vi "Server Client Loop.vi"(0 "Local Hash":string, 3 "Event Logging":refnum<class "EventLoggingService.lvclass">, 4 "Local Version":string, 5 "TCPMessageAPI":refnum<class "TCPMessageAPI.lvclass">, 6 "Client Action Q":refnum<queue>, 7 "Fwd Queue":refnum<queue>, 8 "TCP Client":refnum<k5>, 9 "Remote Port":u16, 10 "Remote Address":string, 11 "Conn Handlers":refnum<queue>) -> ()   [LabVIEW 2020, in "Vecto.lvlib" / "TCPMessaging.lvclass"]
uses:
  TCPMessaging.lvclass
  TX Payload.ctl
  Client Action Data.ctl
  Client Action.ctl
  Client Info.ctl
  TCPMessageService/TCPMessageAPI.lvclass
  proto/TcpClientHello/Data.ctl
  TCPConnectionHandler/TCPConnectionHandler.lvclass
  EventLoggingService/EventLoggingService.lvclass
  Server Client State.ctl
  proto/ConnectStatus/Enumeration.ctl
  Connection State.ctl
  EventLoggingService/EventLoggingService.lvclass/EventLoggingService.ctl
  proto/TcpServerHello/Data.ctl
  EventLogHandler/EventLogHandler.lvclass
  TCPMessaging.lvclass/TCPMessaging.ctl
  Vecto.lvlib
  proto/TcpClientHello/TcpClientHello.lvlib
  VectoConfig/VectoConfig.lvlib
  proto/ConnectStatus/ConnectStatus.lvlib
  proto/TcpServerHello/TcpServerHello.lvlib
panel:
  out "State":T1
  out "Client Hello":T2
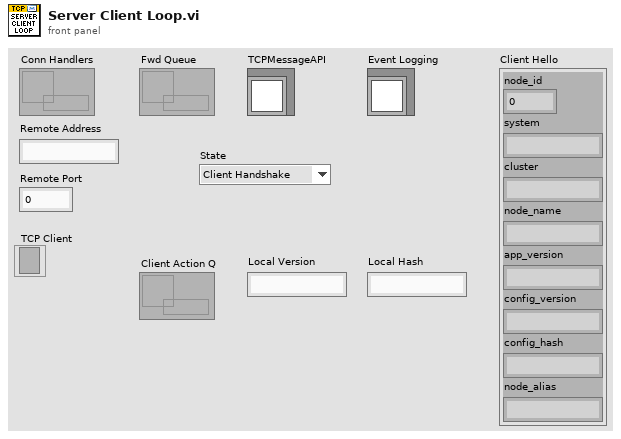
[diagram p1: front panel]
types:
  T1 = typedef "Vecto.lvlib/TCPMessaging.lvclass/Server Client State.ctl" = enum16{"Client Handshake", "Server Handshake", "Message", "Close"}
  T2 = typedef "TcpClientHello.lvlib/Data.ctl" = cluster{"node_id":u32, "system":string, "cluster":string, "node_name":string, "app_version":string, "config_version":string, "config_hash":string, "node_alias":string}
  T3 = enum16{"big-endian, network order", "native, host order", "little-endian"}
  T4 = typedef "ConnectStatus.lvlib/Enumeration.ctl" = enum16{"STATUS_UNKNOWN", "STATUS_SUCCESS", "STATUS_ERROR", "STATUS_BAD_CONFIG", "STATUS_BAD_SYSTEM", "STATUS_BAD_CLUSTER", "STATUS_NOT_ALLOWED"}
  T5 = typedef "Vecto.lvlib/TCPMessaging.lvclass/Client Action.ctl" = enum16{"Connect", "Ready", "Disconnect"}
  T6 = typedef "Vecto.lvlib/TCPMessaging.lvclass/Client Action Data.ctl" = cluster{"Client Action":T5, "Client Info":T7, "TCP":refnum<k5>, "TX Q":refnum<queue>}
  T7 = typedef "VectoConfig.lvlib/Client Info.ctl" = cluster{"TcpClientHello":cluster{"node_id":u32, "system":string, "cluster":string, "node_name":string, "app_version":string, "config_version":string, "config_hash":string, "node_alias":string}, "Remote Address":string, "Remote Port":u16}
  T8 = typedef "Vecto.lvlib/Connection State.ctl" = enum16{"Connected", "Disconnected"}
  T9 = typedef "TcpServerHello.lvlib/Data.ctl" = cluster{"status":T4}
  T10 = typedef "Vecto.lvlib/TX Payload.ctl" = cluster{"Target ID":u32, "Payload":string}
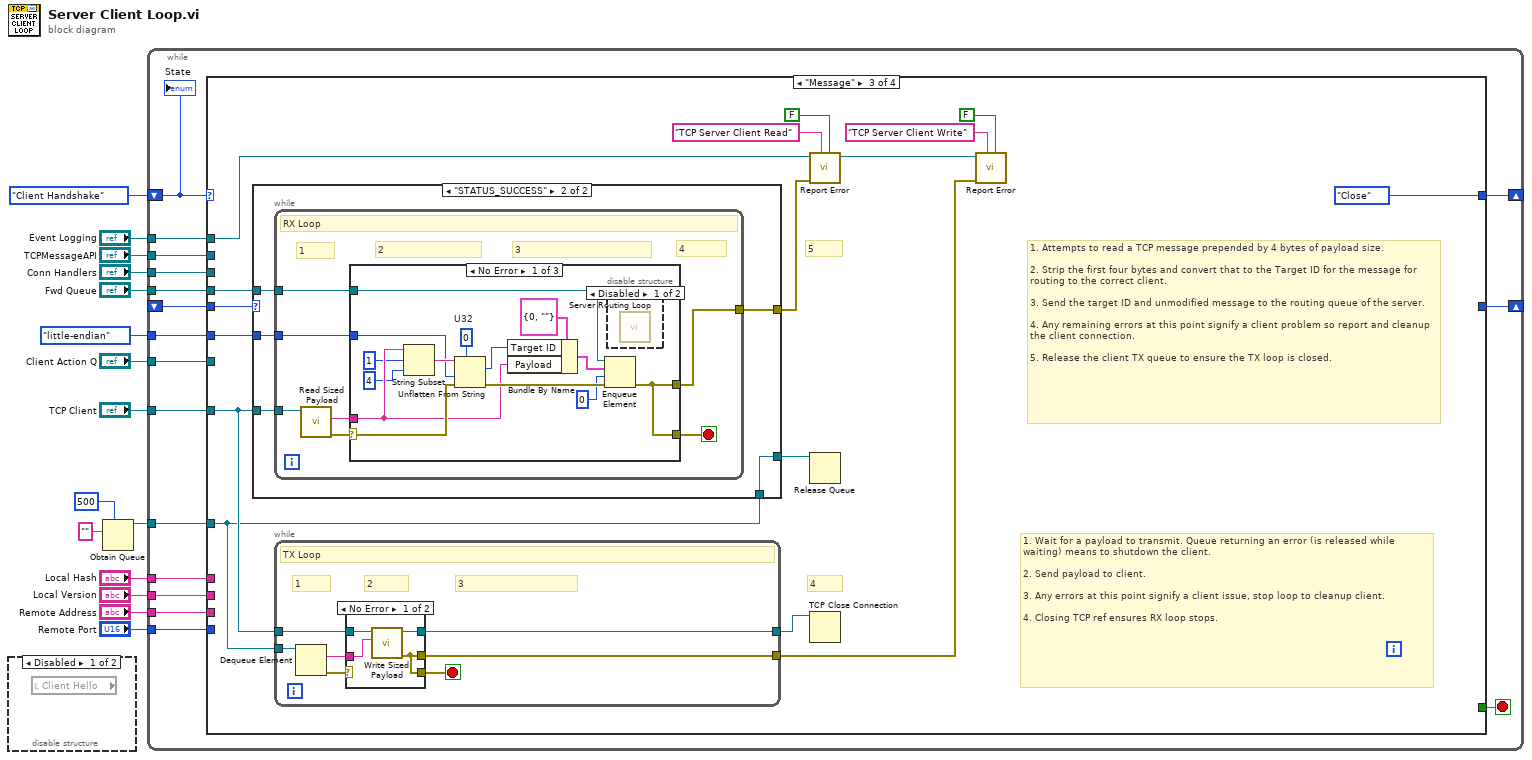
[diagram p0: block diagram]
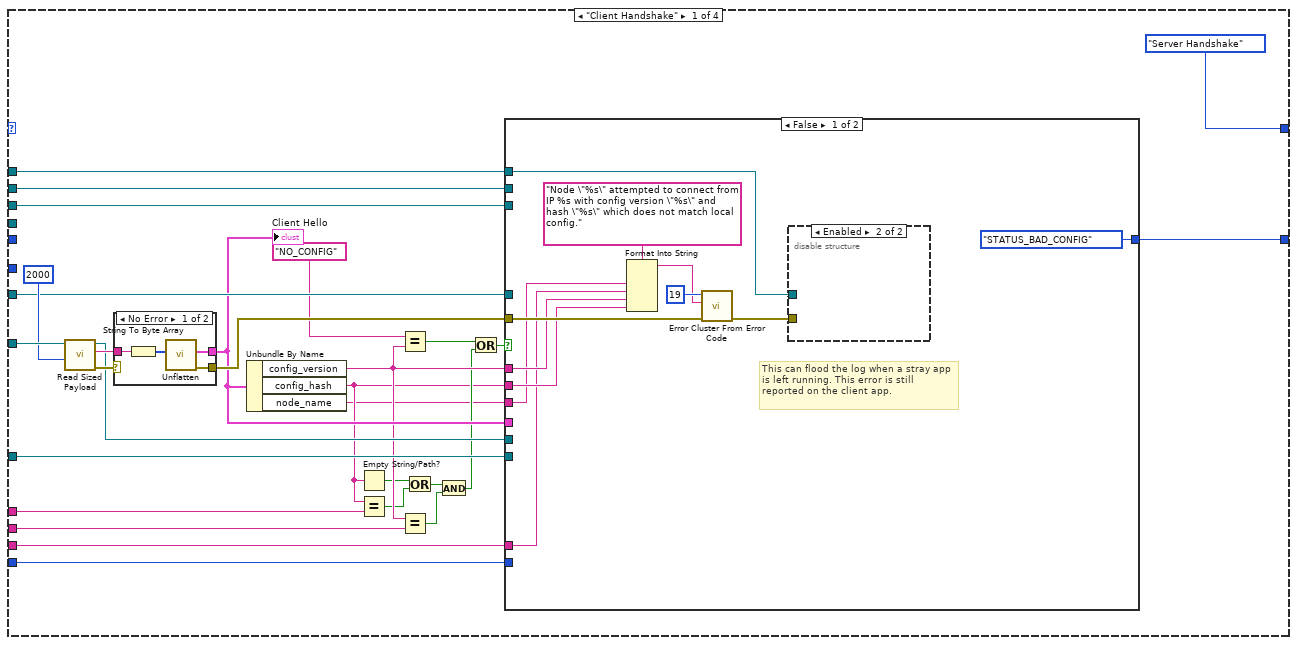
[diagram p2: hidden frame]
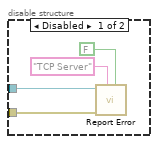
[diagram p3: hidden frame]
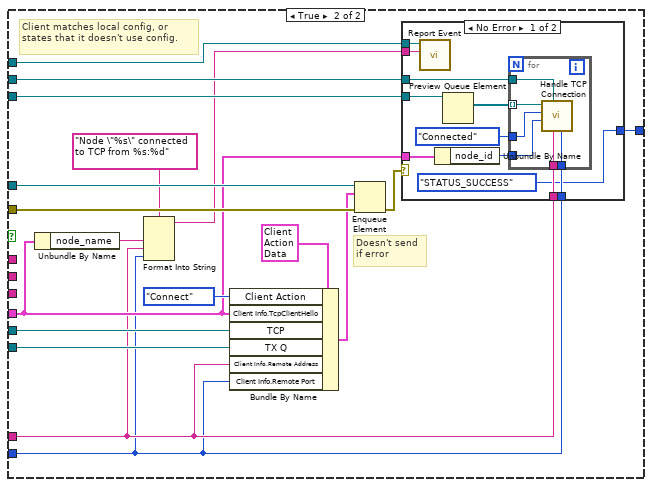
[diagram p4: hidden frame]
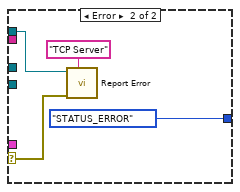
[diagram p5: hidden frame]
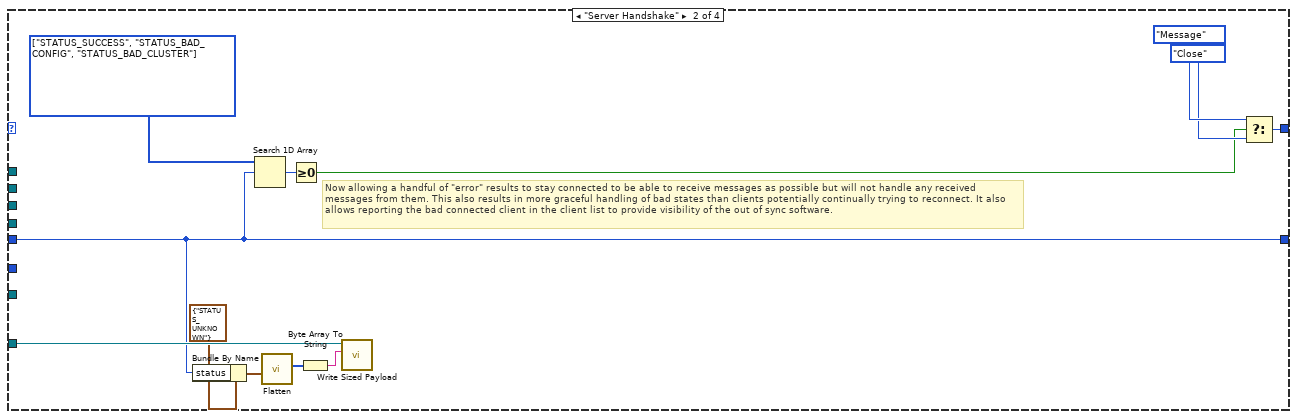
[diagram p7: hidden frame]
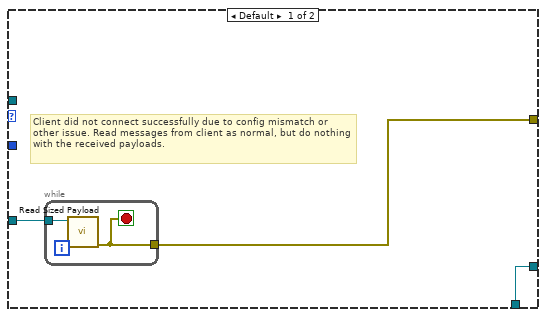
[diagram p8: hidden frame]
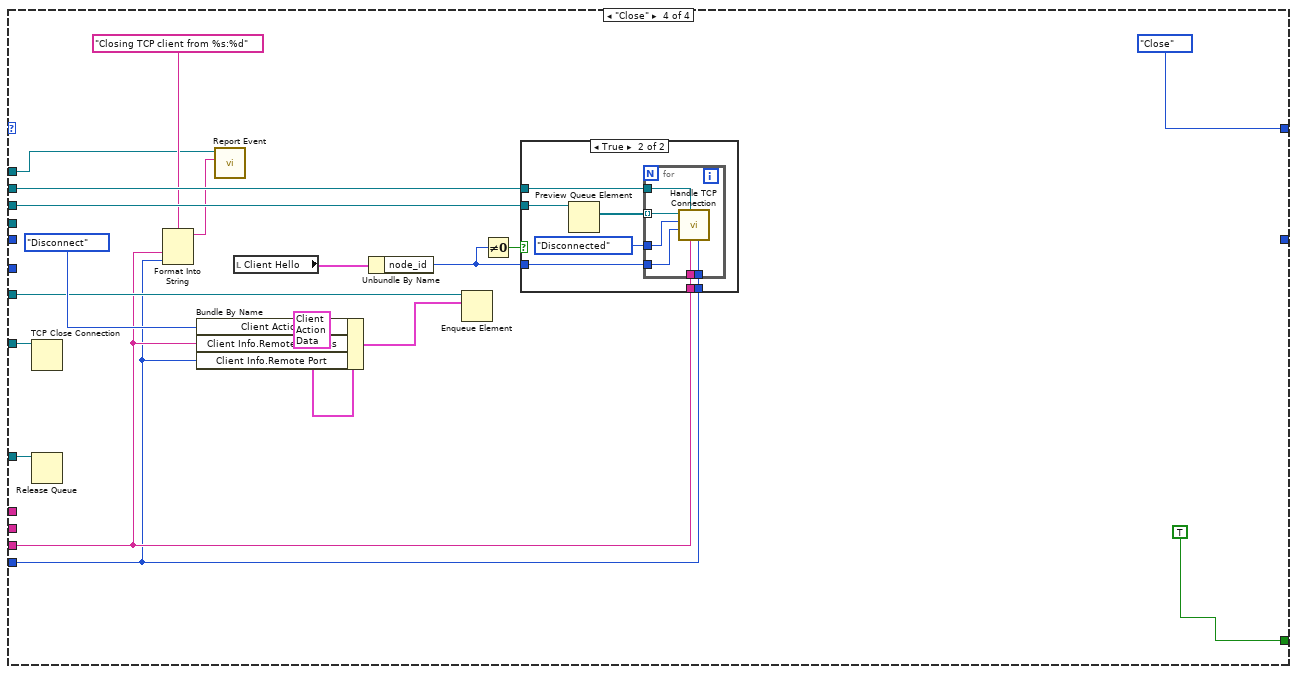
[diagram p13: hidden frame]
diagram:
  n1 = disable-structure shown="Disabled" {
    frame Disabled {
      n2 = local read "Client Hello"() -> ()  [unwired: 1 out]
    }
    frame Enabled {
    }
  }
  n3 = Obtain Queue(max queue size (-1, unlimited)=500, element data type="") -> (queue out=w7:refnum<queue>)  [unwired: 3 in, 2 out]
  n4 = while {
    tunnel: "Fwd Queue" -> [w32]
    tunnel: "TCP Client" -> [w31]
    tunnel: T3."little-endian" ("byte order (0:big-endian, network order)") -> [w30]
    shift-right: [w27] -> _
    shift-left: Server_Client_State."Client Handshake" ("Server Client State") -> [w28]
    tunnel: "Remote Address" -> [w26]
    tunnel: "Remote Port" -> [w25]
    tunnel: w7 -> [w24]
    tunnel: "Client Action Q" -> [w23]
    tunnel: "Conn Handlers" -> [w22]
    tunnel: "TCPMessageAPI" -> [w21]
    tunnel: "Local Version" -> [w20]
    tunnel: "Event Logging" -> [w19]
    shift-right: [w18] -> _
    shift-left: _ -> [w17]
    tunnel: "Local Hash" -> [w16]
    stop <- w29 stop-if-true
    n5 = case shown="\"Message\"" w28 {
      tunnel: w32 -> [_ _ w148 _]
      tunnel: w31 -> [w60 w129 w147 w208]
      tunnel: w30 -> [_ _ w146 _]
      tunnel: [_ _ _ TRUE] -> w29
      tunnel: [Server_Client_State."Server Handshake" ("Server Client State") w130 Server_Client_State."Close" ("Server Client State") Server_Client_State."Close" ("Server Client State")] -> w27
      tunnel: w26 -> [w51 _ _ w198]
      tunnel: w25 -> [w50 _ _ w197]
      tunnel: w24 -> [w54 _ w142 w209]
      tunnel: w23 -> [w56 _ _ w206]
      tunnel: w22 -> [w53 _ _ w203]
      tunnel: w21 -> [w52 _ _ w202]
      tunnel: w20 -> [w48 _ _ _]
      tunnel: w19 -> [w44 _ w139 w195]
      tunnel: [w41 w123 _ _] -> w18
      tunnel: w17 -> [_ w123 w141 _]
      tunnel: w16 -> [w40 _ _ _]
      frame "Client Handshake" {
        n6 = call "Read Sized Payload.vi"("timeout ms (100)"=2000, "TCP in"=w60) -> ("error out"=w58:errorcluster, "Payload"=w57:string, "TCP"=w55:refnum<k5>)  [unwired: 7 in]
        n7 = case shown="No Error" w58 {
          selector: w58 -> [_ w120]
          tunnel: w57 -> [w119 _]
          tunnel: [w117 _] -> w49
          tunnel: [w116 w120] -> w61
          frame No Error {
            n8 = String To Byte Array(string=w119) -> (unsigned byte array=w118:u8[])
            n9 = call "Unflatten.vi"("Buffer"=w118) -> ("error out"=w116:errorcluster, "Data"=w117:T2)  [unwired: 9 in]
          }
          frame Error {
          }
        }
        "Client Hello" <- w49
        n10 = Unbundle By Name(w49) -> ("config_version"=w43:string, "config_hash"=w37:string, "node_name"=w33:string)
        n11 = Empty String/Path?(string/path=w37) -> (empty?=w36:bool)
        n12 = Equal?(x=w37, y=w40) -> (x = y?=w35:bool)
        n13 = Equal?(x="NO_CONFIG", y=w43) -> (x = y?=w46:bool)
        n14 = Equal?(x=w43, y=w48) -> (x = y?=w39:bool)
        n15 = Or(x=w36, y=w35) -> (x .or. y?=w34:bool)
        n16 = And(x=w34, y=w39) -> (x .and. y?=w38:bool)
        n17 = Or(x=w46, y=w38) -> (x .or. y?=w45:bool)
        n18 = case shown="False" w45 {
          tunnel: w61 -> [w72 w93]
          tunnel: w56 -> [_ w92]
          tunnel: w55 -> [_ w89]
          tunnel: w54 -> [_ w87]
          tunnel: w53 -> [_ w86]
          tunnel: w52 -> [_ w85]
          tunnel: w51 -> [w62 w82]
          tunnel: w50 -> [_ w81]
          tunnel: w49 -> [_ w84]
          tunnel: w44 -> [w71 w78]
          tunnel: w43 -> [w68 _]
          tunnel: [Enumeration."STATUS_BAD_CONFIG" ("Enumeration") w77] -> w41
          tunnel: w37 -> [w64 _]
          tunnel: w33 -> [w63 _]
          frame False {
            # "This can flood the log when a stray app is left running. This error is still reported on the client app."
            n19 = Format Into String(format string="Node \"%s\" attempted to connect from IP %s with config version \"%s\" and hash \"%s\" which does not match local config.", w63, w62, w68, w64) -> (resulting string=w67:string)  [unwired: 2 in, 1 out]
            n20 = call <vilib>:"Error Cluster From Error Code.vi"("error in (no error)"=w72, "error message (\"\")"=w67, "error code (0)"=19) -> ("error out"=w66:errorcluster)  [unwired: 6 in]
            n21 = disable-structure shown="Enabled" {
              disable-tunnel: w71 -> [w76 _]
              disable-tunnel: w66 -> [w75 _]
              frame Disabled {
                n22 = call "Report Error.vi"("Callchain (T)"=FALSE, "Context (None)"="TCP Server", "error in (no error)"=w75, "EventLoggingService in"=w76) -> ()  [unwired: 6 in, 2 out]
              }
              frame Enabled {
              }
            }
          }
          frame True {
            # "Client matches local config, or states that it doesn't use config."
            # "Doesn't send if error"
            n23 = Unbundle By Name(w84) -> ("node_name"=w83:string)
            n24 = Format Into String(format string="Node \"%s\" connected to TCP from %s:%d", w83, w82, w81) -> (resulting string=w79:string)  [unwired: 2 in, 1 out]
            n25 = Bundle By Name(cluster=T6 {"Client Action"=enum."Disconnect", "Client Info"={"TcpClientHello"={"node_id"=0, "system"="", "cluster"="", "node_name"="", "app_version"="", "config_version"="", "config_hash"="", "node_alias"=""}, "Remote Address"="", "Remote Port"=0}, "TCP"=refnum, "TX Q"=refnum} ("element"), "Client Action"=Client_Action."Connect", "Client Info.TcpClientHello"=w84, "TCP"=w89, "TX Q"=w87, "Client Info.Remote Address"=w82, "Client Info.Remote Port"=w81) -> (w88:T6)
            n26 = Enqueue Element(queue=w92, element=w88, error in (no error)=w93) -> (error out=w94:errorcluster)  [unwired: 1 in, 2 out]
            n27 = case shown="No Error" w94 {
              selector: w94 -> [_ w114]
              tunnel: w86 -> [w101 _]
              tunnel: w84 -> [w105 _]
              tunnel: w85 -> [w104 _]
              tunnel: w82 -> [w99 _]
              tunnel: w81 -> [w98 _]
              tunnel: w79 -> [w97 _]
              tunnel: w78 -> [w96 w115]
              tunnel: [Enumeration."STATUS_SUCCESS" ("Enumeration") Enumeration."STATUS_ERROR" ("Enumeration")] -> w77
              frame No Error {
                n28 = call "Report Event.vi"("Message"=w97, "EventLoggingService in"=w96) -> ()  [unwired: 8 in, 2 out]
                n29 = Unbundle By Name(w105) -> ("node_id"=w103:u32)
                n30 = Preview Queue Element(queue=w101) -> (element=w100:refnum<class "TCPConnectionHandler.lvclass">[])  [unwired: 2 in, 3 out]
                n31 = for {
                  tunnel: w100 -> [w111] mode=indexing
                  tunnel: w104 -> [w110]
                  tunnel: w103 -> [w108]
                  tunnel: Connection_State."Connected" ("Connection State") -> [w109]
                  tunnel: w99 -> [w107]
                  tunnel: w98 -> [w106]
                  n32 = call-dynamic "Handle TCP Connection.vi"("Remote Port"=w106, "Remote Host"=w107, "TCPMessageAPI"=w110, "Node ID"=w108, "Connection State"=w109, "TCPConnectionHandler in"=w111) -> ()  [unwired: 4 in, 2 out]
                }
              }
              frame Error {
                n33 = call "Report Error.vi"("Context (None)"="TCP Server", "error in (no error)"=w114, "EventLoggingService in"=w115) -> ()  [unwired: 7 in, 2 out]
              }
            }
          }
        }
      }
      frame "Server Handshake" {
        w124 = T4[] [enum."STATUS_SUCCESS", enum."STATUS_BAD_CONFIG", enum."STATUS_BAD_CLUSTER"] items=["STATUS_UNKNOWN", "STATUS_SUCCESS", "STATUS_ERROR", "STATUS_BAD_CONFIG", "STATUS_BAD_SYSTEM", "STATUS_BAD_CLUSTER", "STATUS_NOT_ALLOWED"]
        # "Now allowing a handful of \"error\" results to stay connected to be able to receive messages as possible but will not handle any received messages from them. This also results in more graceful handling of bad states than clients potentially continually trying to reconnect. It also allows reporting the bad connected client in the client list to provide visibility of the out of sync software."
        n34 = Bundle By Name(cluster=T9 {"status"=enum."STATUS_UNKNOWN"} ("Data"), "status"=w123) -> (w125:T9)
        n35 = Search 1D Array(1D array=w124, element=w123) -> (index of element=w122:i32)  [unwired: 1 in]
        n36 = call "Flatten.vi"("Data"=w125) -> ("Buffer"=w128:u8[])  [unwired: 9 in, 1 out]
        n37 = Greater Or Equal To 0?(x=w122) -> (x >= 0?=w121:bool)
        n38 = Byte Array To String(unsigned byte array=w128) -> (string=w127:string)
        n39 = call "Write Sized Payload.vi"("Payload"=w127, "TCP in"=w129) -> ()  [unwired: 8 in, 2 out]
        n40 = Select(t=Server_Client_State."Message" ("Server Client State"), s=w121, f=Server_Client_State."Close") -> (s? t:f=w130:T1)
      }
      frame "Message" {
        # "4"
        # "5"
        # "1. Wait for a payload to transmit. Queue returning an error (is released while waiting) means to shutdown the client.\n\n2. Send payload to client.\n\n3. Any errors at this point signify a client issue, stop loop to cleanup client.\n\n4. Closing TCP ref ensures RX loop stops."
        # "1. Attempts to read a TCP message prepended by 4 bytes of payload size.\n\n2. Strip the first four bytes and convert that to the Target ID for the message for routing to the correct client.\n\n3. Send the target ID and unmodified message to the routing queue of the server.\n\n4. Any remaining errors at this point signify a client problem so report and cleanup the client connection.\n\n5. Release the client TX queue to ensure the TX loop is closed."
        n41 = case shown="\"STATUS_SUCCESS\"" w141 {
          tunnel: w148 -> [_ w158]
          tunnel: w147 -> [w150 w157]
          tunnel: w146 -> [_ w156]
          tunnel: [w151 w155] -> w143
          tunnel: w142 -> [w151 w155]
          tunnel: [w149 w154] -> w140
          frame Default {
            # "Client did not connect successfully due to config mismatch or other issue. Read messages from client as normal, but do nothing with the received payloads."
            n42 = while {
              tunnel: w150 -> [w153]
              tunnel: [w152] -> w149
              stop <- w152 stop-if-true
              n43 = call "Read Sized Payload.vi"("TCP in"=w153) -> ("error out"=w152:errorcluster)  [unwired: 8 in, 2 out]
            }
          }
          frame "STATUS_SUCCESS" {
            n44 = while {
              tunnel: w158 -> [w165]
              tunnel: w157 -> [w163]
              tunnel: w156 -> [w164]
              tunnel: [w159] -> w154
              stop <- w160 stop-if-true
              # "3"
              # "2"
              # "4"
              # "1"
              # "RX Loop"
              n45 = call "Read Sized Payload.vi"("TCP in"=w163) -> ("error out"=w162:errorcluster, "Payload"=w161:string)  [unwired: 8 in, 1 out]
              n46 = case shown="No Error" w162 {
                selector: w162 -> [w179 w180 _]
                tunnel: [w166 w180 _] -> w160
                tunnel: w165 -> [w177 _ _]
                tunnel: w164 -> [w170 _ _]
                tunnel: w161 -> [w169 _ _]
                tunnel: [w166 _ _] -> w159
                frame No Error {
                  w174 = u32 0  # U32
                  n47 = String Subset(string=w169, offset (0)=1 ("length (rest)"), length (rest)=4 ("length (rest)")) -> (substring=w175:string)
                  n48 = Unflatten From String(type=w174, binary string=w175, byte order (0:big-endian, network order)=w170, error in (no error)=w179) -> (value=w172:u32, error out=w178:errorcluster)  [unwired: 1 in, 1 out]
                  n49 = Bundle By Name(cluster=T10 {"Target ID"=0, "Payload"=""} ("TX Payload"), "Target ID"=w172, "Payload"=w169) -> (w171:T10)
                  n50 = Enqueue Element(queue=w177, element=w171, timeout in ms (-1)=0, error in (no error)=w178) -> (error out=w166:errorcluster)  [unwired: 2 out]
                  n51 = disable-structure shown="Disabled" {
                    frame Disabled {
                      n52 = call "Server Routing Loop.vi"() -> ()  [unwired: 11 in, 1 out]
                    }
                    frame Enabled {
                    }
                  }
                }
                frame Default {
                }
                frame Error {
                  # "Timeout, don't propagate error to iterate again and wait another interval for data."
                }
              }
            }
          }
        }
        n53 = while {
          tunnel: w142 -> [w187]
          tunnel: w147 -> [w186]
          tunnel: [w183] -> w145
          tunnel: [w182] -> w133
          stop <- w181 stop-if-true
          # "3"
          # "2"
          # "1"
          # "TX Loop"
          n54 = Dequeue Element(queue=w187) -> (element=w185:string, error out=w184:errorcluster)  [unwired: 2 in, 2 out]
          n55 = case shown="No Error" w184 {
            selector: w184 -> [_ w192]
            tunnel: w186 -> [w190 w193]
            tunnel: w185 -> [w191 _]
            tunnel: [w188 _] -> w182
            tunnel: [w189 w193] -> w183
            tunnel: [w188 w192] -> w181
            frame No Error {
              n56 = call "Write Sized Payload.vi"("Payload"=w191, "TCP in"=w190) -> ("error out"=w188:errorcluster, "TCP"=w189:refnum<k5>)  [unwired: 8 in]
            }
            frame Default {
            }
          }
        }
        n57 = call "Report Error.vi"("Callchain (T)"=FALSE, "Context (None)"="TCP Server Client Read", "error in (no error)"=w140, "EventLoggingService in"=w139) -> ("EventLoggingService out"=w134:refnum<class "EventLoggingService.lvclass">)  [unwired: 6 in, 1 out]
        n58 = Release Queue(queue=w143) -> ()  [unwired: 2 in, 3 out]
        n59 = TCP Close Connection(connection ID=w145) -> ()  [unwired: 2 in, 2 out]
        n60 = call "Report Error.vi"("Callchain (T)"=FALSE, "Context (None)"="TCP Server Client Write", "error in (no error)"=w133, "EventLoggingService in"=w134) -> ()  [unwired: 6 in, 2 out]
      }
      frame "Close" {
        n61 = TCP Close Connection(connection ID=w208) -> ()  [unwired: 2 in, 2 out]
        n62 = Release Queue(queue=w209) -> ()  [unwired: 2 in, 3 out]
        n63 = Format Into String(format string="Closing TCP client from %s:%d", w198, w197) -> (resulting string=w194:string)  [unwired: 2 in, 1 out]
        n64 = Bundle By Name(cluster=T6 {"Client Action"=enum."Disconnect", "Client Info"={"TcpClientHello"={"node_id"=0, "system"="", "cluster"="", "node_name"="", "app_version"="", "config_version"="", "config_hash"="", "node_alias"=""}, "Remote Address"="", "Remote Port"=0}, "TCP"=refnum, "TX Q"=refnum} ("element"), "Client Action"=Client_Action."Disconnect", "Client Info.Remote Address"=w198, "Client Info.Remote Port"=w197) -> (w204:T6)
        n65 = call "Report Event.vi"("Message"=w194, "EventLoggingService in"=w195) -> ()  [unwired: 8 in, 2 out]
        n66 = local read "Client Hello"() -> (w201:T2)
        n67 = Unbundle By Name(w201) -> ("node_id"=w200:u32)
        n68 = Enqueue Element(queue=w206, element=w204) -> ()  [unwired: 2 in, 3 out]
        n69 = Not Equal To 0?(x=w200) -> (x != 0?=w199:bool)
        n70 = case shown="True" w199 {
          tunnel: w203 -> [_ w216]
          tunnel: w202 -> [_ w218]
          tunnel: w200 -> [_ w217]
          tunnel: w198 -> [_ w213]
          tunnel: w197 -> [_ w212]
          frame False {
          }
          frame True {
            n71 = Preview Queue Element(queue=w216) -> (element=w215:refnum<class "TCPConnectionHandler.lvclass">[])  [unwired: 2 in, 3 out]
            n72 = for {
              tunnel: w218 -> [w224]
              tunnel: w217 -> [w223]
              tunnel: w215 -> [w222] mode=indexing
              tunnel: Connection_State."Disconnected" ("Connection State") -> [w221]
              tunnel: w213 -> [w220]
              tunnel: w212 -> [w219]
              n73 = call-dynamic "Handle TCP Connection.vi"("Remote Port"=w219, "Remote Host"=w220, "TCPMessageAPI"=w224, "Node ID"=w223, "Connection State"=w221, "TCPConnectionHandler in"=w222) -> ()  [unwired: 4 in, 2 out]
            }
          }
        }
      }
    }
    "State" <- w28
  }
